vi "Write ESPAÑOL.vi"(8 "error in (no error)":errorcluster, 10 "ESPAÑOL":bool, 11 "CAFE ACTOR in":refnum<class "CAFE ACTOR.lvclass">) -> (0 "error out":errorcluster, 3 "CAFE ACTOR out":refnum<class "CAFE ACTOR.lvclass">)   [LabVIEW 2019, in "CAFE ACTOR.lvlib" / "CAFE ACTOR.lvclass"]
uses:
  CAFE ACTOR.lvclass
  CAFE ACTOR.lvclass/CAFE ACTOR.ctl
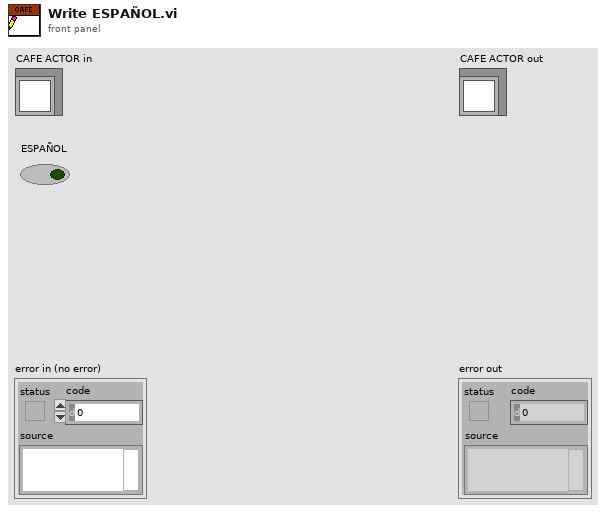
[diagram p1: front panel]
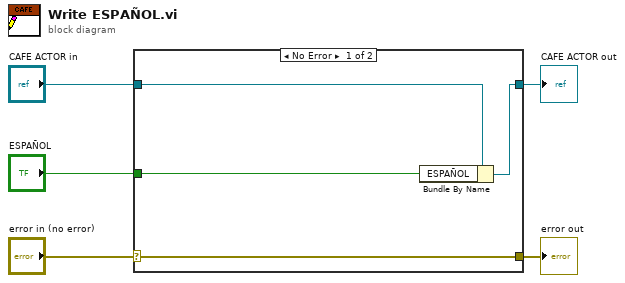
[diagram p0: block diagram]
diagram:
  n1 = case shown="No Error" "error in (no error)" {
    selector: "error in (no error)" -> [w9 w10]
    tunnel: [w9 w10] -> w4
    tunnel: [w7 w11] -> w2
    tunnel: "CAFE ACTOR in" -> [w8 w11]
    tunnel: "ESPAÑOL" -> [w6 _]
    frame No Error {
      n2 = Bundle By Name(cluster=w8, "ESPAÑOL"=w6) -> (w7:refnum<class "CAFE ACTOR.lvclass">)
    }
    frame Error {
    }
  }
  "error out" <- w4
  "CAFE ACTOR out" <- w2
